vi "get_fast_cmd_settings.vi"(7 "Settings in":string) -> (0 "*WAI":bool, 1 "OPC?":bool, 2 "ErrorCheckMode":i32, 3 "DataType":i32)   [LabVIEW 2014, in "rszvl_rsidr_core.lvlib"]
uses:
  rszvl_rsidr_core.lvlib
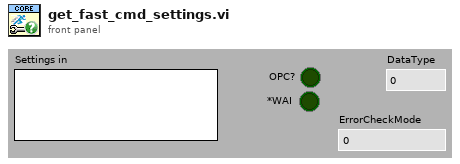
[diagram p1: front panel]
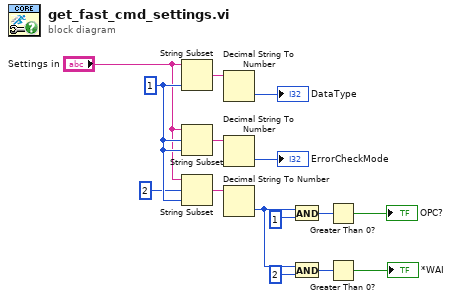
[diagram p0: block diagram]
diagram:
  w10 = 1 ("length (rest)")
  n1 = String Subset(string="Settings in", length (rest)=w10) -> (substring=w15:string)  [unwired: 1 in]
  n2 = String Subset(string="Settings in", offset (0)=w10, length (rest)=w10) -> (substring=w13:string)
  n3 = String Subset(string="Settings in", offset (0)=2, length (rest)=w10) -> (substring=w11:string)
  n4 = Decimal String To Number(string=w15) -> (number=→"DataType":i32)  [unwired: 2 in, 1 out]
  n5 = Decimal String To Number(string=w13) -> (number=→"ErrorCheckMode":i32)  [unwired: 2 in, 1 out]
  n6 = Decimal String To Number(string=w11) -> (number=w1:i32)  [unwired: 2 in, 1 out]
  n7 = And(x=w1, y=1) -> (x .and. y?=w6:i32)
  n8 = And(x=w1, y=2) -> (x .and. y?=w4:i32)
  n9 = Greater Than 0?(x=w6) -> (x > 0?=→"OPC?":bool)
  n10 = Greater Than 0?(x=w4) -> (x > 0?=→"*WAI":bool)
